vi "Write Pattern Data 2.vi"(8 "error in (no error)":errorcluster, 10 "Pattern Data":T2={"Name"="", "Litho"=[], "Set Resistance"=enum."1G ohm", "Meta"=variant}, 11 "AFM_Driver in":refnum<class "AFM_Driver.lvclass">) -> (0 "error out":errorcluster, 3 "AFM_Driver out":refnum<class "AFM_Driver.lvclass">)   [LabVIEW 2019, in "AFM_Driver.lvclass"]
uses:
  AFM_Driver.lvclass
  <userlib>/LevyLab/Relay Box/Typedefs/Resistor--enum.ctl
  AFM_Driver.lvclass/AFM_Driver.ctl
  <userlib>/LevyLab/Relay Box/Relay-Box.lvclass
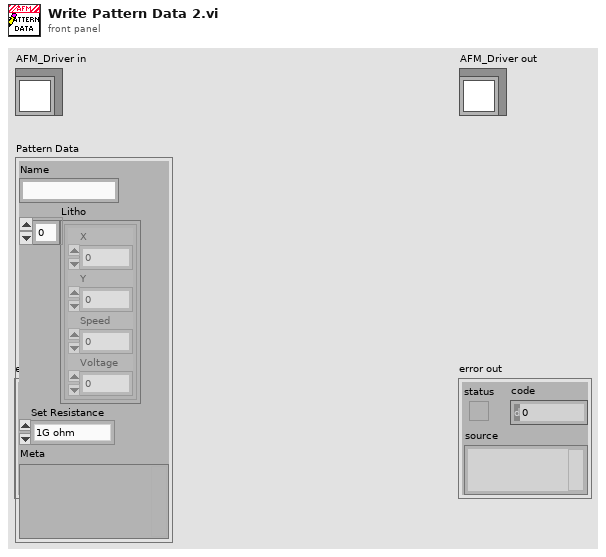
[diagram p1: front panel]
types:
  T1 = typedef "Relay-Box.lvclass/Resistor--enum.ctl" = enum16{"open", "discharge tip", "0 ohms", "100k ohm", "10M ohm", "1G ohm"}
  T2 = cluster{"Name":string, "Litho":cluster{"X":dbl, "Y":dbl, "Speed":dbl, "Voltage":dbl}[], "Set Resistance":T1, "Meta":variant}
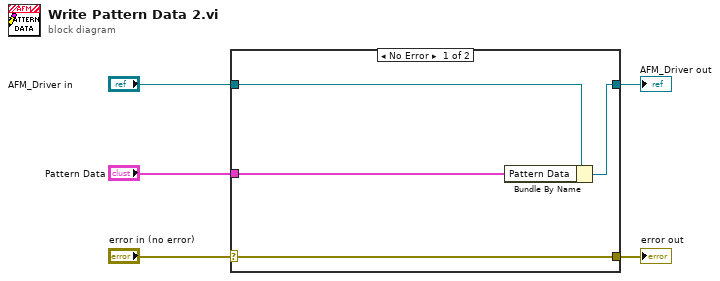
[diagram p0: block diagram]
diagram:
  n1 = case shown="No Error" "error in (no error)" {
    selector: "error in (no error)" -> [w9 w10]
    tunnel: [w9 w10] -> w4
    tunnel: [w7 w11] -> w2
    tunnel: "AFM_Driver in" -> [w8 w11]
    tunnel: "Pattern Data" -> [w6 _]
    frame No Error {
      n2 = Bundle By Name(cluster=w8, "Pattern Data"=w6) -> (w7:refnum<class "AFM_Driver.lvclass">)
    }
    frame Error {
    }
  }
  "error out" <- w4
  "AFM_Driver out" <- w2
